vi "String.Split to Lines.vi"(11 "String":string) -> (2 "Count":i32, 3 "Lines":string[](array[string]))   [LabVIEW 2018]
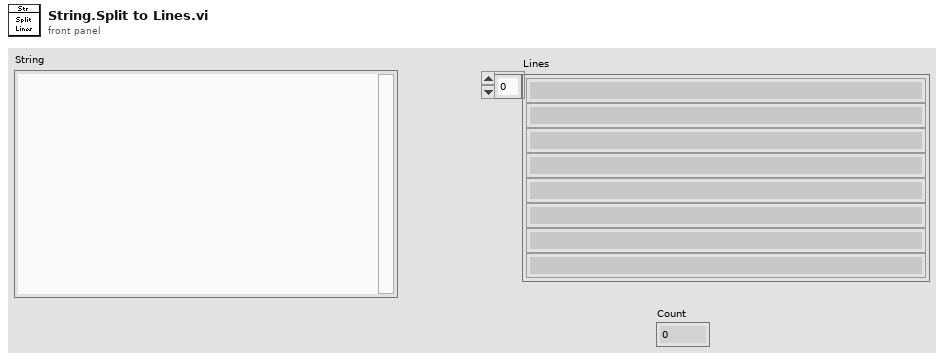
[diagram p1: front panel]
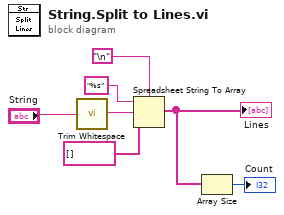
[diagram p0: block diagram]
diagram:
  n1 = call <vilib>:"Trim Whitespace.vi"("string"="String") -> ("trimmed string"=w6:string)  [unwired: 1 in]
  n2 = Spreadsheet String To Array(delimiter (Tab)="\n", format string="%s", spreadsheet string=w6, array type (2D Dbl)=string[] []) -> (array=w1:string[])
  "Lines" <- w1
  n3 = Array Size(array=w1) -> (size(s)=→"Count":i32)
